vi "Excit_Process_Wfm.vi"(4 "Excit Form":T1(ring)=enum."Swift", 5 "Factor":dbl=0.8 format="%#_13g", 6 "Duration (µs)":dbl=800.0, 7 "Sampling Frequency (MHz)":dbl=20.0, 8 "End Frequency (kHz)":dbl=250.0, 9 "Start Frequency (kHz)":dbl=250.0, 10 "Amplitude (%)":dbl=100.0) -> (0 "FFT Excitation":dbl[](array[numeric]), 1 "X Freq":dbl[](array[numeric]), 2 "Signal Excitation":dbl[](array[numeric]), 3 "X Time":dbl[](array[numeric]))   [LabVIEW 2017]
doc: "From a start and end value, generates an adiabatic waveform signal of 2000 values (double).\nWrites this waveform into a binary file, in a big-endian format.\nDisplays the written data and the FFT of the signal.\nDefault Path for the generated file is D:\\PIRENEA\\EXCIT_WFMS\n\nAvailable Waveforms : Sinus, Swift, Chirp, Ramp (Up or Down), DoubleRamp (Up-Down or Down-Up)"
uses:
  <vilib>/Analysis/2dsp.llb/Inverse Complex FFT.vi
  <vilib>/Analysis/NI_AALPro.lvlib
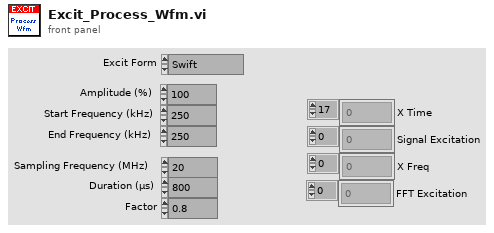
[diagram p1: front panel]
types:
  T1 = enum16{"Sinus", "Chirp", "Swift", "TwoSwift", "Ramp"}
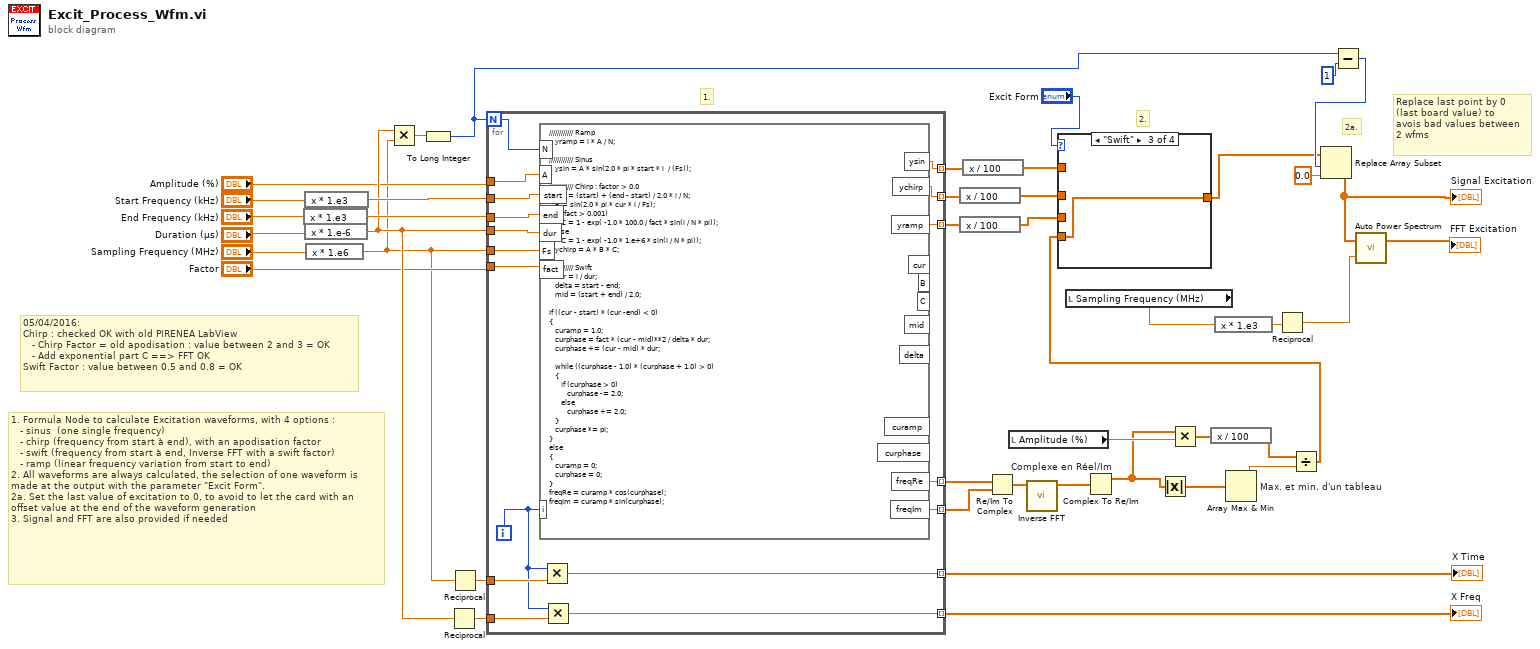
[diagram p0: block diagram]
diagram:
  # "Replace last point by 0\n(last board value) to\navois bad values between\n2 wfms"
  # "2a."
  # "2."
  # "05/04/2016:\nChirp : checked OK with old PIRENEA LabView\n   - Chirp Factor = old apodisation : value between 2 and 3 = OK\n   - Add exponential part C ==> FFT OK\nSwift Factor : value between 0.5 and 0.8 = OK"
  # "1."
  # "1. Formula Node to calculate Excitation waveforms, with 4 options :\n   - sinus  (one single frequency)\n   - chirp (frequency from start à end), with an apodisation factor\n   - swift (frequency from start à end, Inverse FFT with a swift factor)\n   - ramp (linear frequency variation from start to end)\n2. All waveforms are always calculated, the selection of one waveform is made at the output with the parameter \"Excit Form\".\n2a. Set the last value of excitation to 0, to avoid to let the card with an offset value at the end of the waveform generation\n3. Signal and FFT are also provided if needed"
  n1 = expression code="x * 1.e3"("End Frequency (kHz)") -> (w42:dbl)
  n2 = expression code="x * 1.e3"("Start Frequency (kHz)") -> (w43:dbl)
  n3 = expression code="x * 1.e-6"("Duration (µs)") -> (w23:dbl)
  n4 = expression code="x * 1.e6"("Sampling Frequency (MHz)") -> (w3:dbl)
  n5 = Multiply(x=w23, y=w3) -> (x*y=w35:dbl)
  n6 = To Long Integer(number=w35) -> (32bit integer=w8:i32)
  n7 = Reciprocal(x=w23) -> (1/x=w22:dbl)
  n8 = Reciprocal(x=w3) -> (1/x=w24:dbl)
  n9 = for {
    N: w8 -> [w60]
    tunnel: [w59] -> w32 mode=indexing
    tunnel: w42 -> [w55]
    tunnel: [w58] -> w34 mode=indexing
    tunnel: w43 -> [w56]
    tunnel: "Amplitude (%)" -> [w57]
    tunnel: w23 -> [w53]
    tunnel: w3 -> [w54]
    tunnel: [w52] -> w39 mode=indexing
    tunnel: [w51] -> w38 mode=indexing
    tunnel: "Factor" -> [w50]
    tunnel: [w49] -> w28 mode=indexing
    tunnel: w24 -> [w48]
    tunnel: [w47] -> w25 mode=indexing
    tunnel: w22 -> [w45]
    tunnel: [w44] -> w21 mode=indexing
    i -> [w46]
    n10 = formula code="//////////// Ramp\n   yramp = i * A / N;\n\n//////////// Sinus\n   ysin = A * sin(2.0 * pi * start * i  / (Fs));\n\n//////////// Chirp : factor > 0.0\n   cur = (start) + (end - start) / 2.0 * i / N;\n   B = sin(2.0 * pi * cur * i / Fs);\n   if (fact > 0.001)\n      C = 1 - exp( -1.0 * 100.0 / fact * sin(i / N * pi));\n   else\n      C = 1 - exp( -1.0 * 1.e+6 * sin(i / N * pi));\n   ychirp = A * B * C;\n   \n//////////// Swift\n   cur = i / dur;\n   delta = start - end;\n   mid = (start + end) / 2.0;\n\nif ((cur - start) * (cur -end) < 0)\n{\n   curamp = 1.0;\n   curphase = fact * (cur - mid)**2 / delta * dur;\n   curphase += (cur - mid) * dur;\n\n   while ((curphase - 1.0) * (curphase + 1.0) > 0)\n   {\n      if (curphase > 0)\n         curphase -= 2.0;\n      else\n         curphase += 2.0;\n   }\n   curphase *= pi;\n}\nelse\n{\n   curamp = 0;\n   curphase = 0;\n}\nfreqRe = curamp * cos(curphase);\nfreqIm = curamp * sin(curphase);"("A"=w57, "start"=w56, "i"=w46, "N"=w60, "end"=w55, "Fs"=w54, "dur"=w53, "fact"=w50) -> ("ychirp"=w59:dbl, "ysin"=w58:dbl, "freqRe"=w52:dbl, "freqIm"=w51:dbl, "yramp"=w49:dbl)  [unwired: 7 out]
    n11 = Multiply(x=w46, y=w48) -> (x*y=w47:dbl)
    n12 = Multiply(x=w46, y=w45) -> (x*y=w44:dbl)
  }
  "X Time" <- w25
  "X Freq" <- w21
  n13 = expression code="x / 100"(w32) -> (w31:dbl[])
  n14 = expression code="x / 100"(w28) -> (w27:dbl[])
  n15 = expression code="x / 100"(w34) -> (w33:dbl[])
  n16 = Re/Im To Complex(1:w38, 2:w39) -> (0:w37:cdb[])
  n17 = local read "Amplitude (%)"() -> (w26:dbl)
  n18 = call-poly <vilib>:"Inverse FFT.vi"("FFT {X}"=w37) -> ("X"=w40:cdb[])  [unwired: 9 in, 1 out]
  n19 = local read "Sampling Frequency (MHz)"() -> (w4:dbl)
  n20 = Complex To Re/Im "Complexe en Réel/Im"(x + iy=w40) -> (x=w2:dbl[])  [unwired: 1 out]
  n21 = Absolute Value(x=w2) -> (abs(x)=w1:dbl[])
  n22 = Multiply(x=w2, y=w26) -> (x*y=w30:dbl[])
  n23 = expression code="x / 100"(w30) -> (w29:dbl[])
  n24 = expression code="x * 1.e3"(w4) -> (w19:dbl)
  n25 = Array Max & Min "Max. et min. d'un tableau"(array=w1) -> (max value=w41:dbl)  [unwired: 3 out]
  n26 = Reciprocal(x=w19) -> (1/x=w20:dbl)
  n27 = Divide(x=w29, y=w41) -> (x/y=w36:dbl[])
  n28 = case shown="\"Swift\"" "Excit Form" {
    tunnel: [w61 w62 w63 w64] -> w6
    tunnel: w36 -> [_ _ w63 _]
    tunnel: w33 -> [w61 _ _ _]
    tunnel: w31 -> [_ w62 _ _]
    tunnel: w27 -> [_ _ _ w64]
    frame "Sinus", Default {
    }
    frame "Chirp" {
    }
    frame "Swift" {
    }
    frame "Ramp" {
    }
  }
  n29 = Subtract(x=w8, y=1) -> (x-y=w7:i32)
  n30 = Replace Array Subset(array=w6, new element=0.0 ("nouvel élément/sous-tableau"), index=w7) -> (w5:dbl[])
  "Signal Excitation" <- w5
  n31 = call <vilib>:"Auto Power Spectrum.vi"("dt"=w20, "Signal (V)"=w5) -> ("Power Spectrum (V^2 rms)"=→"FFT Excitation":dbl[])  [unwired: 1 out]
